vi "OldIntakeNetwork.vi"(8 "error in (no error)":errorcluster) -> (0 "error out":errorcluster)   [LabVIEW 2023]
uses:
  OldIntakeGlobal.vi
  <vilib>/Rock Robotics/Network Tables/NT Write Number.vi
  <vilib>/Rock Robotics/Network Tables/NT Write Boolean.vi
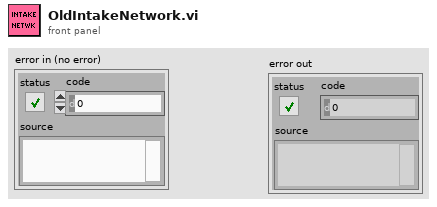
[diagram p1: front panel]
types:
  T1 = typedef "OldIntakeState.ctl" = enum16{"0-init", "1-cancel", "2-wait-for-cmd", "3-intake-check-for-note", "4-intake-start-intake", "5-intake-have-note-yet", "6-intake-stop-motor", "7-spit-out", "8-feed-note-to-shooter"}
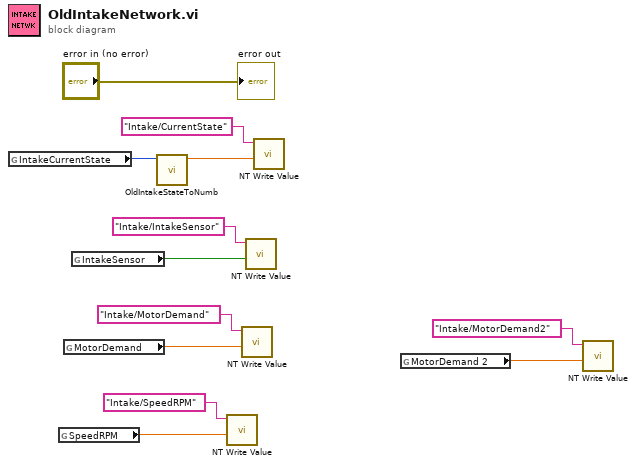
[diagram p0: block diagram]
diagram:
  n1 = global read "OldIntakeGlobal.vi" "IntakeCurrentState"() -> (w4:T1)
  n2 = global read "OldIntakeGlobal.vi" "SpeedRPM"() -> (w11:dbl)
  n3 = global read "OldIntakeGlobal.vi" "MotorDemand"() -> (w6:dbl)
  n4 = global read "OldIntakeGlobal.vi" "IntakeSensor"() -> (w8:bool)
  n5 = call "OldIntakeStateToNumb.vi"("Intake_State"=w4) -> ("StateNumber"=w3:dbl)  [unwired: 10 in]
  n6 = call-poly <vilib>:"NT Write Value.vi"("value"=w11, "name"="Intake/SpeedRPM") -> ()  [unwired: 9 in, 1 out]
  n7 = call-poly <vilib>:"NT Write Value.vi"("value"=w6, "name"="Intake/MotorDemand") -> ()  [unwired: 9 in, 1 out]
  n8 = call-poly <vilib>:"NT Write Value.vi"("value"=w8, "name"="Intake/IntakeSensor") -> ()  [unwired: 9 in, 1 out]
  n9 = call-poly <vilib>:"NT Write Value.vi"("value"=w3, "name"="Intake/CurrentState") -> ()  [unwired: 9 in, 1 out]
  n10 = global read "OldIntakeGlobal.vi" "MotorDemand 2"() -> (w1:dbl)
  n11 = call-poly <vilib>:"NT Write Value.vi"("value"=w1, "name"="Intake/MotorDemand2") -> ()  [unwired: 9 in, 1 out]
  "error out" <- "error in (no error)"
